vi "show_last_Foto.vi"(8 "error in (no error)":T1, 11 "Carpeta":path=path "C:/Imagenes/experimentos") -> (0 "error":T1)   [LabVIEW 2017]
panel:
  out "Error":bool
  out "Running":bool
  out "Resized Picture":picture
  in  "Power On Button":bool
  out "#Foto":dbl
  out "ultimaFoto":path
  # "Lector de la última imagen"
  # "asslcdms Feb2023 LV17"
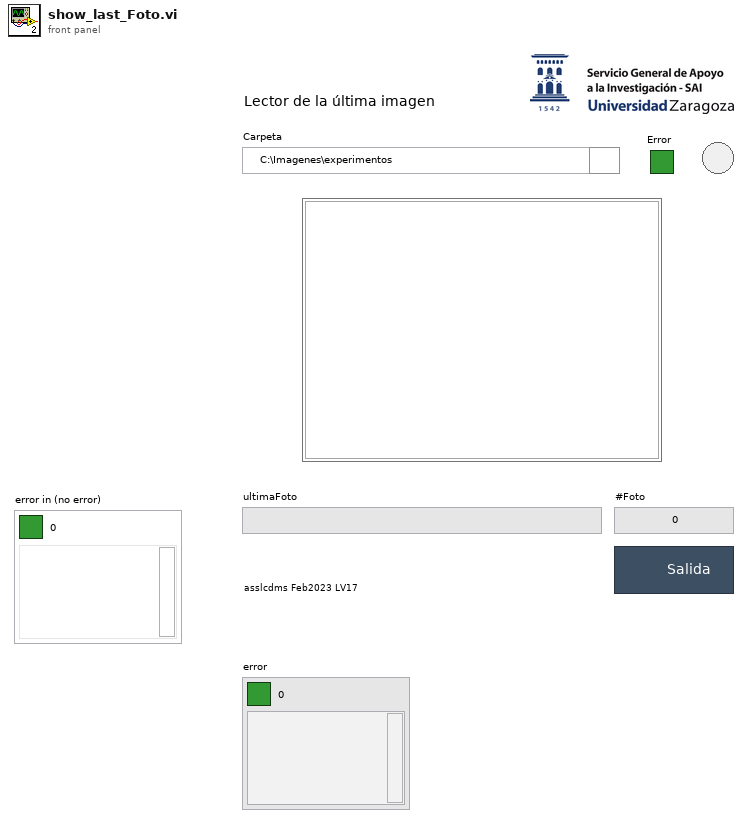
[diagram p1: front panel]
types:
  T1 = cluster{"Boolean Round":bool, "code":i32, "source":string}
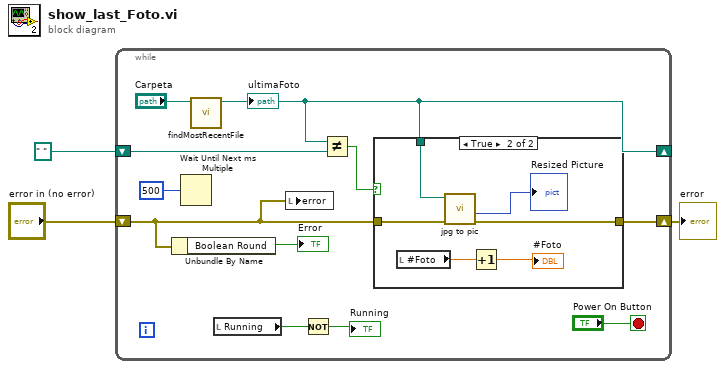
[diagram p0: block diagram]
diagram:
  n1 = while {
    shift-right: [w11] -> _
    shift-left: path " " ("File Path Out") -> [w13]
    shift-right: [w8] -> w1
    shift-left: "error in (no error)" -> [w5]
    stop <- "Power On Button" stop-if-true
    n2 = Unbundle By Name(w5) -> ("Boolean Round"=→"Error":bool)
    n3 = Wait Until Next ms Multiple(millisecond multiple=u32 500) -> ()  [unwired: 1 out]
    n4 = call "findMostRecentFile.vi"("Folder Path In"="Carpeta") -> ("File Path Out"=w11:path)  [unwired: 9 in, 1 out]
    "ultimaFoto" <- w11
    n5 = local read "Running"() -> (w7:bool)
    n6 = local write "error"(w5) -> ()
    n7 = Not(x=w7) -> (.not. x?=→"Running":bool)
    n8 = Not Equal?(x=w11, y=w13) -> (x != y?=w12:bool)
    n9 = case shown="True" w12 {
      tunnel: w11 -> [_ w21]
      tunnel: w5 -> [w15 w18]
      tunnel: [w15 w17] -> w8
      frame False {
      }
      frame True {
        n10 = local read "#Foto"() -> (w20:dbl)
        n11 = call "jpg to pic.vi"("error in (no error)"=w18, "path to JPEG file"=w21) -> ("error out"=w17:errorcluster, "Resized Picture"=→"Resized Picture":picture)  [unwired: 8 in]
        n12 = Increment(x=w20) -> (x+1=→"#Foto":dbl)
      }
    }
  }
  "error" <- w1
